vi "Gyro PID Back Color Assisted.vi"(6 "Target angle":sgl, 7 "Threshold to Stop":i32=1200, 8 "Threshold to slow":i32=1000, 9 "Min. speed":i32=40, 10 "Max. speed":i32=80, 11 "EV3 in":T1) -> (3 "EV3 out":T1)   [LabVIEW 2016]
uses:
  <vilib>/NXT/Subs/LVHSConnector.ctl
  <vilib>/NXT/LegoClasses/BrickReference/BrickReference.lvclass
  <vilib>/NXT/Block Support/NXT_OutputPort.ctl
  <vilib>/NXT/Block Support/NXT_InputPort.ctl
  <vilib>/NXT/NXTIO Xnodes/NXTIONodeSubVIs/LEGOResetMotors.vi
  <vilib>/NXT/Dual Mode Library/Motors/Rotation.vi
  <vilib>/NXT/Dual Mode Library/Sensors/EV3_Color_Reflect.vi
  <vilib>/NXT/NXTIO Xnodes/NXTIONodeSubVIs/NXTMotorSteeringOn.vi
  <vilib>/NXT/NXTIO Xnodes/NXTIONodeSubVIs/NXTStopMotors.vi
  <vilib>/NXT/Dual Mode Library/Waits/Wait_Num.vi
  <vilib>/NXT/NXTIO Xnodes/NXTIOXNode/NXTIO.xnode
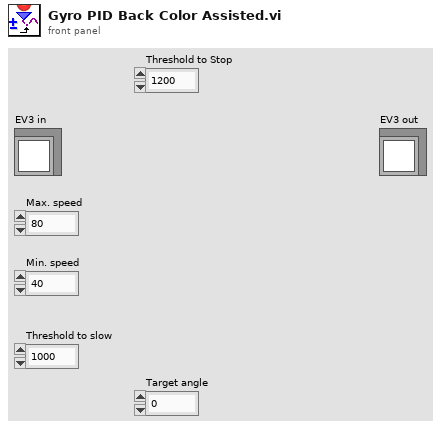
[diagram p1: front panel]
types:
  T1 = typedef "LVHSConnector.ctl" = refnum<class "BrickReference.lvclass">
  T2 = typedef "NXT_OutputPort.ctl" = u8
  T3 = typedef "NXT_InputPort.ctl" = u32
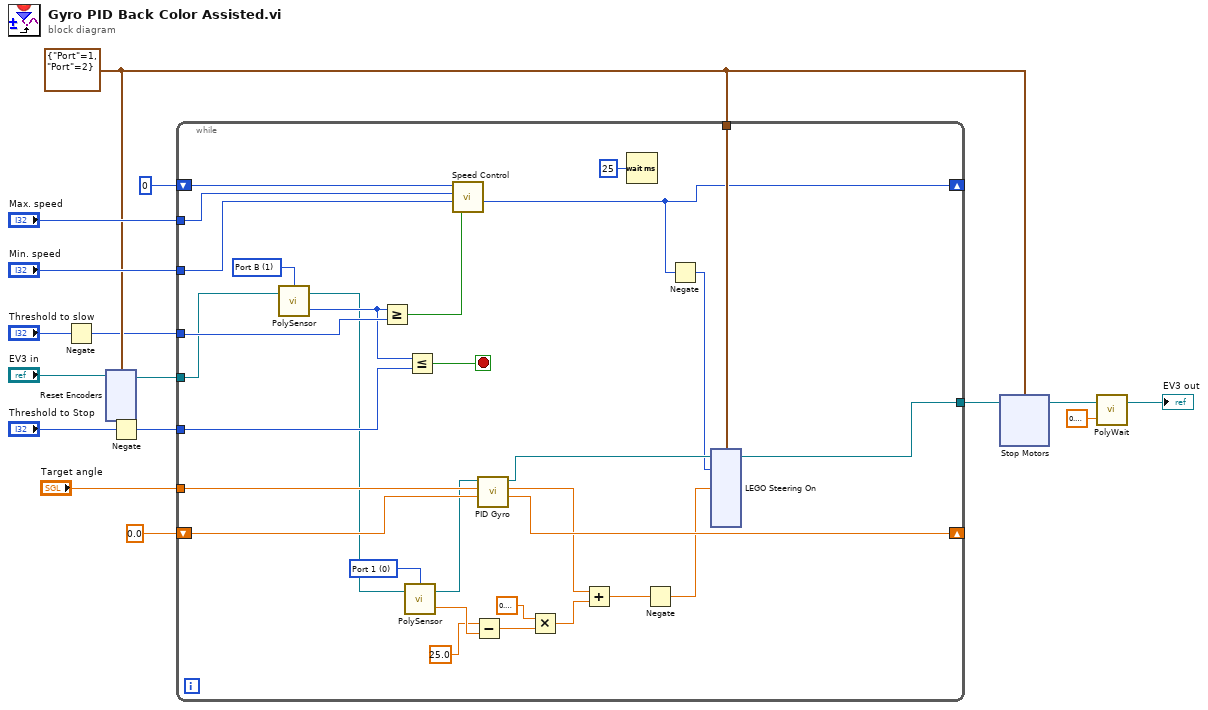
[diagram p0: block diagram]
diagram:
  w6 = cluster{"Port":T2, "Port":T2} {"Port"=1, "Port"=2} ("Motor")
  n1 = Negate(x="Threshold to slow") -> (-x=w2:i32)
  n2 = xnode "Reset Encoders"("Motors"=w6, "NXT/EV3"="EV3 in") -> ("NXT/EV3"=w12:T1)
  n3 = Negate(x="Threshold to Stop") -> (-x=w1:i32)
  n4 = while {
    tunnel: w12 -> [w36]
    shift-right: [w46] -> _
    shift-left: sgl 0.0 -> [w33]
    tunnel: "Target angle" -> [w45]
    tunnel: [w42] -> w8
    tunnel: w6 -> [w44]
    shift-right: [w32] -> _
    shift-left: 0 -> [w40]
    tunnel: "Min. speed" -> [w37]
    tunnel: "Max. speed" -> [w39]
    tunnel: w2 -> [w38]
    tunnel: w1 -> [w31]
    stop <- w19 stop-if-true
    w30 = T3 0 items=["Port 1", "Port 2", "Port 3", "Port 4"] ("Port (Port 1)")
    w43 = T2 1 items=["Port A", "Port B", "Port C", "Port D"] ("Port (Port A)")
    n5 = call-poly <vilib>:"PolySensor.vi"("NXT/EV3"=w36, "Port (Port A)"=w43) -> ("Angle of Rotation"=w34:i32, "NXT/EV3"=w29:T1)  [unwired: 1 in]
    n6 = Greater Or Equal?(x=w34, y=w38) -> (x >= y?=w35:bool)
    n7 = call-poly <vilib>:"PolySensor.vi"("NXT/EV3"=w29, "Port (Port 1)"=w30) -> ("Scaled Value"=w22:sgl, "NXT/EV3"=w28:T1)  [unwired: 1 in]
    n8 = Less Or Equal?(x=w34, y=w31) -> (x <= y?=w19:bool)
    n9 = call "Speed Control.vi"("Speed Up or Down?"=w35, "Min. speed"=w37, "Max. speed"=w39, "Ini. speed"=w40) -> ("Speed out"=w32:i32)  [unwired: 7 in]
    n10 = Subtract(x=sgl 25.0 ("y"), y=w22) -> (x-y=w27:sgl)
    n11 = call "PID Gyro.vi"("Previous integral"=w33, "Target angle"=w45, "EV3 in"=w28) -> ("New integral"=w46:sgl, "Total error"=w24:sgl, "EV3 out"=w20:T1)  [unwired: 6 in]
    n12 = Multiply(x=sgl 0.3, y=w27) -> (x*y=w25:sgl)
    n13 = Add(x=w24, y=w25) -> (x+y=w23:sgl)
    n14 = Wait (ms)(milliseconds to wait=u32 25) -> ()  [unwired: 1 out]
    n15 = Negate(x=w23) -> (-x=w17:sgl)
    n16 = Negate(x=w32) -> (-x=w18:i32)
    n17 = xnode "LEGO Steering On"("Steering 1"=w17, "Power 1"=w18, "Motors"=w44, "NXT/EV3"=w20) -> ("NXT/EV3"=w42:T1)
  }
  n18 = xnode "Stop Motors"("Motors"=w6, "NXT/EV3"=w8) -> ("NXT/EV3"=w7:T1)
  n19 = call-poly <vilib>:"PolyWait.vi"("Time (1 sec)"=sgl 0.2, "NXT/EV3"=w7) -> ("NXT/EV3"=→"EV3 out":T1)  [unwired: 2 in]
